vi "Great little Filter.vi"() -> ()   [LabVIEW 2009]
uses:
  <vilib>/ptbypt/NI_PtbyPt.lvlib
panel:
  out "In":dbl(knob)=0.165419862799715 scale=0.0..1.0
  out "Chan 1":dbl=0.165419862799715
  out "Out":dbl(knob)=0.165419862799715 scale=0.0..1.0
  in  "stop":bool
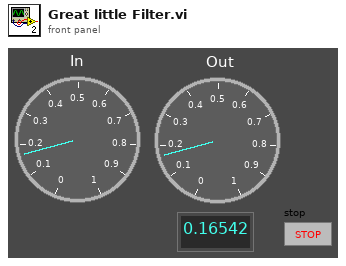
[diagram p1: front panel]
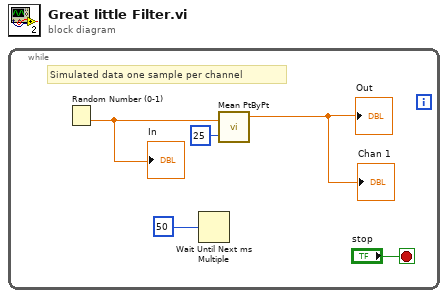
[diagram p0: block diagram]
diagram:
  n1 = while {
    stop <- "stop" stop-if-true
    # "Simulated data one sample per channel"
    n2 = Random Number (0-1)() -> (number: 0 to 1=w1:dbl)
    "In" <- w1
    n3 = Wait Until Next ms Multiple(millisecond multiple=50) -> ()  [unwired: 1 out]
    n4 = call <vilib>:"Mean PtByPt.vi"("x"=w1, "sample length"=25) -> ("mean"=→"Out" →"Chan 1":dbl)  [unwired: 1 in, 2 out]
  }
